vi "Selftest Device Core.vi"(8 "error in (no error)":errorcluster, 11 "LS218 in":refnum<class "LS218.lvclass">) -> (0 "error out":errorcluster, 1 "Self-Test Result Message":string, 2 "Self-Test Result Code":i32, 3 "LS218 out":refnum<class "LS218.lvclass">)   [LabVIEW 2013, in "LS218.lvlib" / "LS218.lvclass"]
doc: "Perform selftest of device."
uses:
  LS218.lvclass
  CSPP_Core/Actors/CS++DeviceActor/CS++DeviceActor.lvclass
  LS218.lvclass/LS218.ctl
  <instrlib>/Lake Shore Cryotronics 218/Lake Shore Cryotronics 218.lvlib
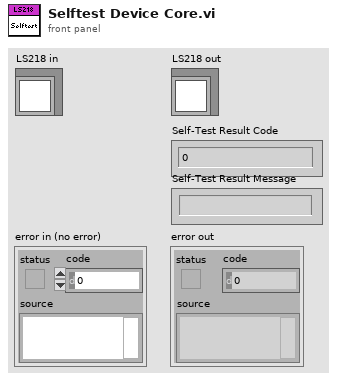
[diagram p1: front panel]
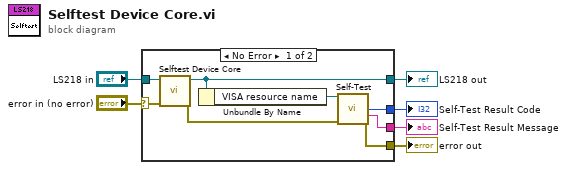
[diagram p0: block diagram]
diagram:
  n1 = case shown="No Error" "error in (no error)" {
    selector: "error in (no error)" -> [w7 w15]
    tunnel: "LS218 in" -> [w14 w16]
    tunnel: [w12 w16] -> w5
    tunnel: [w10 _] -> w4
    tunnel: [w9 _] -> w3
    tunnel: [w8 w15] -> w2
    frame No Error {
      n2 = call-parent "Selftest Device Core.vi"("error in (no error)"=w7, "CS++DeviceActor in"=w14) -> ("error out"=w13:errorcluster, "CS++DeviceActor out"=w12:refnum<class "LS218.lvclass">)  [unwired: 6 in, 2 out]
      n3 = Unbundle By Name(w12) -> ("VISA resource name"=w11:refnum<visa-resource-name>)
      n4 = call <instrlib>:"Self-Test.vi"("VISA resource name"=w11, "error in (no error)"=w13) -> ("Self-Test Error"=w10:u32, "Self-Test Response"=w9:string, "error out"=w8:errorcluster)  [unwired: 10 in, 1 out]
    }
    frame Error {
    }
  }
  "error out" <- w2
  "LS218 out" <- w5
  "Self-Test Result Code" <- w4
  "Self-Test Result Message" <- w3
